vi "GetEnumerator.vi"(8 "error in (no error)":errorcluster caption="错误输入（无错误）", 11 "Queue 输入":refnum<class "Queue.lvclass"> caption="DNL_LabVIEW Object in") -> (0 "error out":errorcluster caption="错误输出", 2 "Enumerator 输出":refnum<class "Enumerator.lvclass">, 3 "Queue 输出":refnum<class "Queue.lvclass"> caption="DNL_LabVIEW Object out")   [LabVIEW 2012, in "Queue.lvclass"]
uses:
  Queue.lvclass
  Enumerator/Enumerator.lvclass
  Queue.lvclass/Queue.ctl
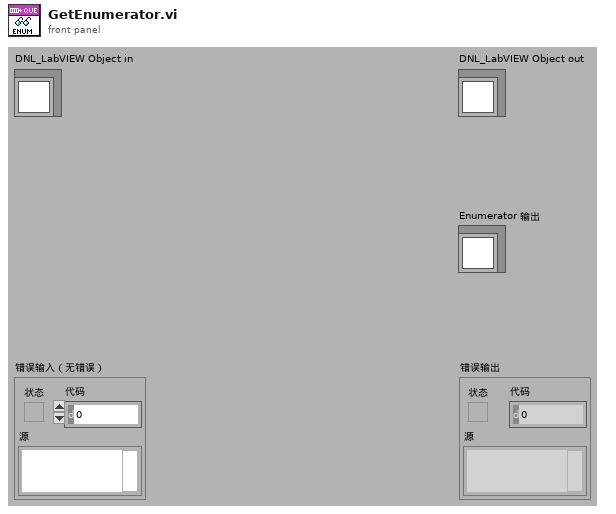
[diagram p1: front panel]
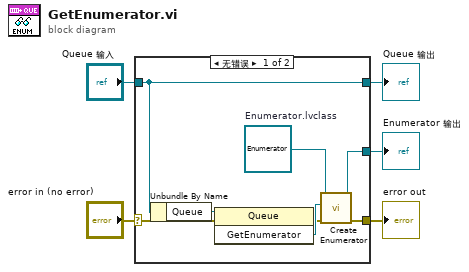
[diagram p0: block diagram]
diagram:
  n1 = case shown="无错误" "error in (no error)" {
    selector: "error in (no error)" -> [w9 w15]
    tunnel: [w7 w15] -> w4
    tunnel: [w12 w14] -> w2
    tunnel: "Queue 输入" -> [w12 w14]
    tunnel: [w6 _] -> w1
    frame No Error {
      w11 = refnum<class "Enumerator.lvclass"> refnum  # Enumerator.lvclass
      n2 = Unbundle By Name(w12) -> ("Queue"=w13:refnum<k24>)
      n3 = invoke class="Queue" method="GetEnumerator"(reference=w13, error in=w9) -> (error out=w8:errorcluster, "GetEnumerator"=w10:refnum<k24>)  [unwired: 1 in, 1 out]
      n4 = call "Create Enumerator.vi"("error in (no error)"=w8, "Enumerator"=w10, "Enumerator 输入"=w11) -> ("error out"=w7:errorcluster, "Enumerator 输出"=w6:refnum<class "Enumerator.lvclass">)  [unwired: 7 in]
    }
    frame Error {
    }
  }
  "error out" <- w4
  "Queue 输出" <- w2
  "Enumerator 输出" <- w1
